vi "Graph - Multi-Y.vi"() -> ()   [LabVIEW 2013, in "Workspace MultiY Graph.lvlib"]
doc: "Sample numeric display item."
uses:
  Workspace MultiY Graph.lvlib
  <vilib>/NI Veristand/Display Template Support/Display Template Support.llb/cluster_Screen Item Settings.ctl
  <vilib>/NI Veristand/Display Template Support/Display Template Support.llb/cluster_Graph Scale Settings.ctl
  <vilib>/NI Veristand/Display Template Support/Display Template Support.llb/cluster_Graph Plot Settings.ctl
  NationalInstruments.VeriStand.SystemStorage
  XY Top level workspace graph data.ctl
  <vilib>/NI Veristand/Execution/Workspace/SystemStateRegEventRef.ctl
  <vilib>/NI Veristand/Display Template Support/Display Template Support.llb/enum_Display Template Handler Minimal To Widget Msg.ctl
  XY Dialog Msg to Control.ctl
  XY Dialog Msg Type.ctl
  XY Persistent Data.ctl
  XY Graph Properties.ctl
  XY Plot Properties.ctl
  XY Scale Properties.ctl
  XY Scale Precision.ctl
  XY Scale Format.ctl
  UDP Data.ctl
  Update Rate.ctl
  XY References.ctl
  <vilib>/NI Veristand/Display Template Support/Display Template Support.llb/enum_Display Template Handler Minimal To Workspace.ctl
  <vilib>/NI Veristand/Execution/Workspace/WorkspaceAPI.ctl
  <vilib>/NI Veristand/Execution/Workspace/SystemStateEventRef.ctl
  XY Control Msg to Dialog.ctl
  <vilib>/NI Veristand/UI Controls/Tree and Alias Browser/Net Event Data Ref.ctl
  <vilib>/NI Veristand/UI Controls/Tree and Alias Browser/Net Event Data.ctl
  <vilib>/NI Veristand/UI Controls/Tree and Alias Browser/Net Event.ctl
  <vilib>/NI Veristand/Execution/Workspace/UDPChannelStreamSession.ctl
  UDP Queue Data.ctl
  UDP Action State.ctl
  Graph Update Queue Data.ctl
  Graph Update Action State.ctl
  UDP Stream Configuration.ctl
  <vilib>/NI Veristand/Execution/Workspace/SystemState.ctl
  <vilib>/Utility/tcp.llb/UDP Multicast Read-Only Open.vi
  <vilib>/NI Veristand/Execution/Workspace/NI_VS Workspace ExecutionAPI.lvlib
  NationalInstruments.VeriStand.ClientAPI
  <vilib>/NI Veristand/UI Controls/Tree and Alias Browser/NI_VS UI Tree Alias Browser.lvlib
panel:
  in  "NIVS.Workspace Event":refnum<event-registration>
  in  "NIVS.System Definition Root":refnum<k24>
  in  "NIVS.Gateway IP Address":string
  out "Label":string="Waveform Graph"
  out "Graph":cluster{"X":dbl[], "Y":dbl[]}[](graph)
  in  "Item.Data":T1
  out "Y.Autoscale":bool
  in  "Y.Scale.Once":bool
  in  "Y.Scale.Auto":bool
  out "X.Autoscale":bool
  in  "X.Scale.Once":bool
  in  "X.Scale.Auto":bool
  in  "Legend":bool
  in  "Setup":bool
  in  "Hold":bool
  # "Autoscale X"
  # "Autoscale Y"
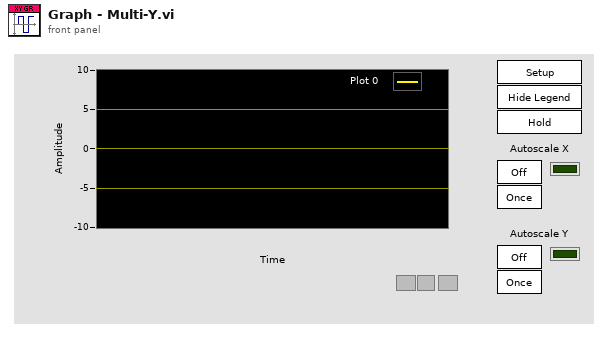
[diagram p1: front panel]
types:
  T1 = typedef "cluster_Screen Item Settings.ctl" = cluster{"Template VI":string, "Position X":i32, "Position Y":i32, "Custom":string, "Show Title Bar":bool, "ID":i32, "Always On Top":bool, "Allow Resize":bool, "Allow Minimize":bool, "Allow Close":bool, "Size to Screen":bool, "Screen.ID":i32, "State":enum16{"Normal", "New"}, "Title":string, "Window Bounds":cluster{"[0]":i16, "[1]":i16, "[2]":i16, "[3]":i16}, "Channel Ref":u64, "Unit":string, "Default Units?":bool, "Flash Limit?":bool, "Color 1":u32, "Color 2":u32, "Color 3":u32, "Color 4":u32, "Bck Color":u32, "Fore Color":u32, "Limit 1":dbl, "Limit 2":dbl, "Limit 3":dbl, "Limit 4":dbl, "Limit Mode 1":i32, "Limit Mode 2":i32, "Limit Mode 3":i32, "Limit Mode 4":i32, "Scale Precision":i32, "Scale Min":dbl, "Scale Max":dbl, "Format":i32, "Precision":i32, "Background Type":i32, "IDs":i32[], "Units":string[], "Labels":string[], "Scale Factor":dbl, "Scale Offset":dbl, "YScale Index":u32[], "XScale":T2, "YScales":T2[], "Plots":T3[], "Update Period":dbl, "History Length":dbl, "My.Ref":refnum<vi>, "Is Control?":bool, "Channel Paths":string[], "Custom Data":variant}
  T2 = typedef "cluster_Graph Scale Settings.ctl" = cluster{"Format":u8, "Precision":u8, "Fit":u8, "Label":string, "Use Default Label":bool, "Label Visible":bool, "Min":dbl, "Max":dbl}
  T3 = typedef "cluster_Graph Plot Settings.ctl" = cluster{"Bar Style":u8, "Fill To":i16, "Fill/PtColor":u32, "Line Style":u8, "Line Width":u8, "Color":u32, "Interp":u8, "Point Style":u8}
  T4 = typedef "Workspace MultiY Graph.lvlib/UDP Action State.ctl" = enum16{"Idle", "Open", "Acquire", "Send", "Close"}
  T5 = typedef "Workspace MultiY Graph.lvlib/UDP Stream Configuration.ctl" = cluster{"net address":u32, "Port":u16, "Channel IDs":i32[], "Packet IDs":i32[], "max packet size":i32, "Graph Buffer Size":i32, "Decimation":i32, "UDP Buffer Size":u32}
  T6 = cluster{"connection ID":refnum<k16>, "UDP Stream Configuration":T5, "Graph Buffer":cluster{"X":dbl[], "Y":dbl[]}[], "Dynamic VI Refs":refnum<vi>[]}
  T7 = typedef "Workspace MultiY Graph.lvlib/Graph Update Action State.ctl" = enum16{"Active", "Change Rate", "Inactive"}
  T8 = typedef "Workspace MultiY Graph.lvlib/Graph Update Queue Data.ctl" = cluster{"Graph Update Action State":T7, "Data":variant}
  T9 = typedef "Workspace MultiY Graph.lvlib/UDP Queue Data.ctl" = cluster{"UDP Action State":T4, "Data":variant}
  T10 = typedef "Workspace MultiY Graph.lvlib/XY Top level workspace graph data.ctl" = cluster{"Custom Data":variant, "EventRegs":cluster{"SystemChange":T11, "WorkspaceState":refnum<event-registration>, "Graph":refnum<event-registration>, "Wks&Dialog&Periodic":refnum<event-registration>}, "References":T12, "Persistent Data":T13, "System":cluster{"To Workspace":refnum<user-event>, "From Workspace":refnum<user-event>, "NIVS helper":refnum<vi>, "Gtwy":string, "Root":refnum<k24>, "Workspace":T21, "SystemStateRefs":T22, "Connected?":bool, "FromDialog":refnum<user-event>, "ErrFlag":bool, "New":bool, "ErrState":string, "Save":bool, "Hold":bool, "Periodic":refnum<user-event>, "ToDialog":refnum<user-event>, "DialogEventReg":refnum<event-registration>, "UseSavedWidth":bool, "TreeBrowserEventReg":refnum<event-registration>, "UDPChannelStreamSession":T23, "Valid Channels?":bool, "Update Graph":refnum<user-event>, "UDP Queue":refnum<queue>, "Graph Update Queue":refnum<queue>}, "GraphData":cluster{"X":dbl[], "Y":dbl[]}[], "UDP Stream Active?":bool}
  T11 = typedef "NI_VS Workspace ExecutionAPI.lvlib/SystemStateRegEventRef.ctl" = refnum<event-registration>
  T12 = typedef "Workspace MultiY Graph.lvlib/XY References.ctl" = cluster{"X.Scale.Auto":refnum<vi>, "Y.Scale.Auto":refnum<vi>, "X.Scale.Once":refnum<vi>, "Y.Scale.Once":refnum<vi>, "LegendVis":refnum<vi>, "Graph":refnum<vi>}
  T13 = typedef "Workspace MultiY Graph.lvlib/XY Persistent Data.ctl" = cluster{"Label":string, "Graph Props":T14, "UDP Data":T19}
  T14 = typedef "Workspace MultiY Graph.lvlib/XY Graph Properties.ctl" = cluster{"Plots":T15[], "Legend:Number of Rows":u32, "Scale Properties":T16, "Legend:Visible":bool, "BgColor":u32, "Last Plot Width":u32, "Resize":bool}
  T15 = typedef "Workspace MultiY Graph.lvlib/XY Plot Properties.ctl" = cluster{"Bar Plot Style":u8, "Digital Line Style":u8, "Digital Transition Location":u8, "Digital Transition Type":u8, "Fill To":i16, "Fill/Point Color":u32, "Label Format":u8, "Line Style":u8, "Line Width":u8, "Plot Color":u32, "Plot Interpolation":u8, "Point Style":u8, "Visible":bool, "X Scale Index":u32, "Y Scale Index":u32}
  T16 = typedef "Workspace MultiY Graph.lvlib/XY Scale Properties.ctl" = cluster{"X.Auto":bool, "X.Min":dbl, "X.Max":dbl, "X.IgnoreTS":bool, "X.Precision":T17, "X.Label:":string, "X.LabelVis":bool, "X.DefLabel":bool, "Y.Auto":bool, "Y.Min":dbl, "Y.Max":dbl, "Y.Format":T18, "Y.Precision:":T17, "Y.Label:":string, "Y.LabelVis":bool, "Y.DefLabel":bool, "X.Format":T18}
  T17 = typedef "Workspace MultiY Graph.lvlib/XY Scale Precision.ctl" = u8
  T18 = typedef "Workspace MultiY Graph.lvlib/XY Scale Format.ctl" = u8
  T19 = typedef "Workspace MultiY Graph.lvlib/UDP Data.ctl" = cluster{"Decimation":i32, "UDP Buffer Size":u32, "History Length":dbl, "Update Rate":T20, "Channel Paths":string[], "Channel Names":string[]}
  T20 = typedef "Workspace MultiY Graph.lvlib/Update Rate.ctl" = enum8{"15 Hz", "10 Hz", "5 Hz", "4 Hz", "3 Hz", "2 Hz", "1 Hz", "0.5 Hz"}
  T21 = typedef "NI_VS Workspace ExecutionAPI.lvlib/WorkspaceAPI.ctl" = refnum<k24>
  T22 = typedef "NI_VS Workspace ExecutionAPI.lvlib/SystemStateEventRef.ctl" = cluster{"CustDatRef":refnum<user-event>, "EvtRef":refnum<k27>}
  T23 = typedef "NI_VS Workspace ExecutionAPI.lvlib/UDPChannelStreamSession.ctl" = refnum<k24>
  T24 = cluster{"connection ID":refnum<k16>, "UDP Stream Configuration out":T5, "Array Out":cluster{"X":dbl[], "Y":dbl[]}[], "Dynamic VI Refs":refnum<vi>[]}
  T25 = typedef "Workspace MultiY Graph.lvlib/XY Control Msg to Dialog.ctl" = enum16{"Stop", "Connecting", "Disconnecting"}
  T26 = typedef "enum_Display Template Handler Minimal To Workspace.ctl" = cluster{"Operation":enum16{"SetCustomData", "DeleteItem"}, "Data":variant}
  T27 = cluster{"SystemChange":T11, "WorkspaceState":refnum<event-registration>, "Graph":refnum<event-registration>, "Wks&Dialog&Periodic":refnum<event-registration>}
  T28 = typedef "enum_Display Template Handler Minimal To Widget Msg.ctl" = enum16{"Stop", "LaunchConfigDialog"}
  T29 = typedef "Workspace MultiY Graph.lvlib/XY Dialog Msg Type.ctl" = enum16{"Update", "Delete"}
  T30 = typedef "NI_VS Workspace ExecutionAPI.lvlib/SystemState.ctl" = u8
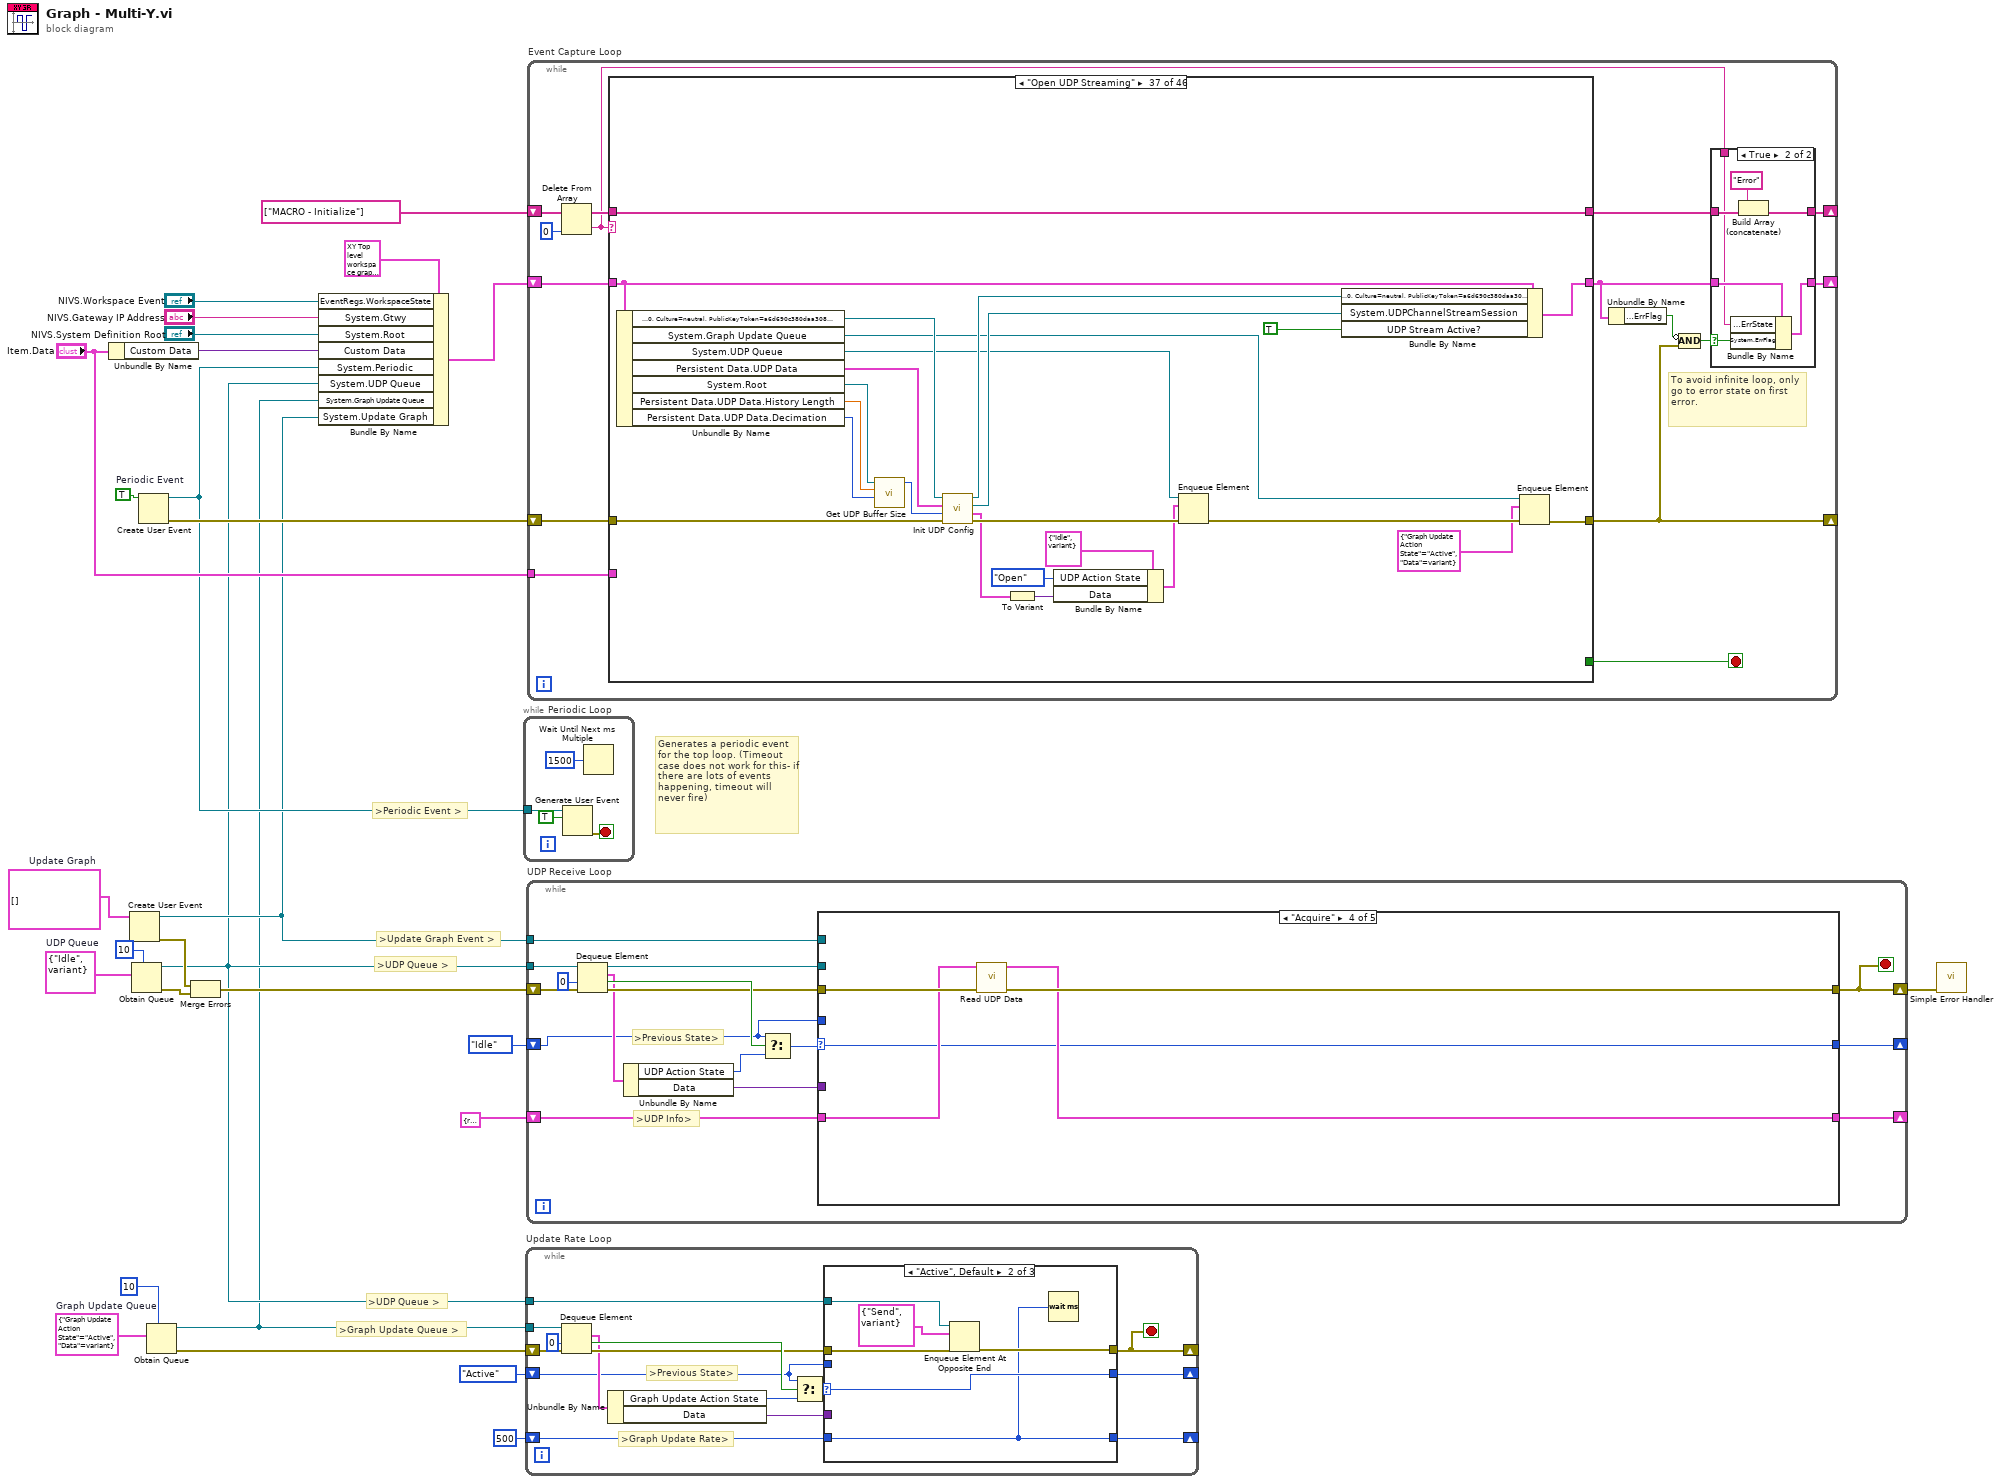
[diagram p0: block diagram]
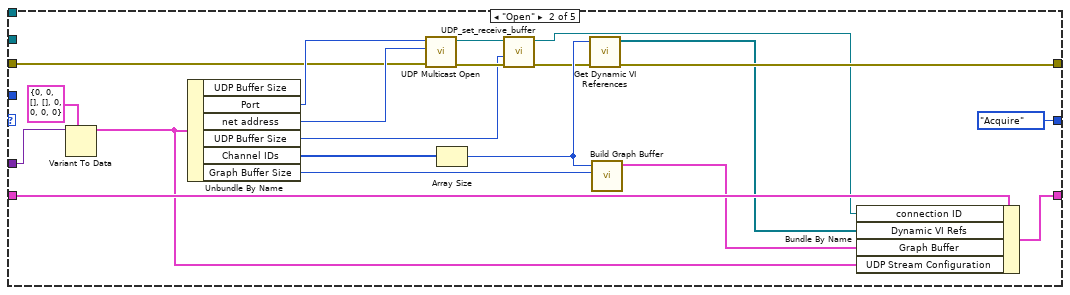
[diagram p3: hidden frame]
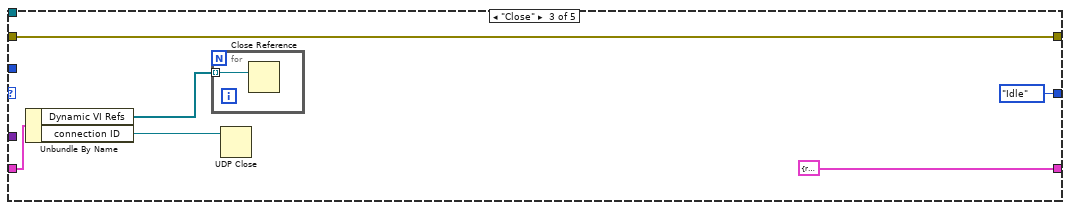
[diagram p4: hidden frame]
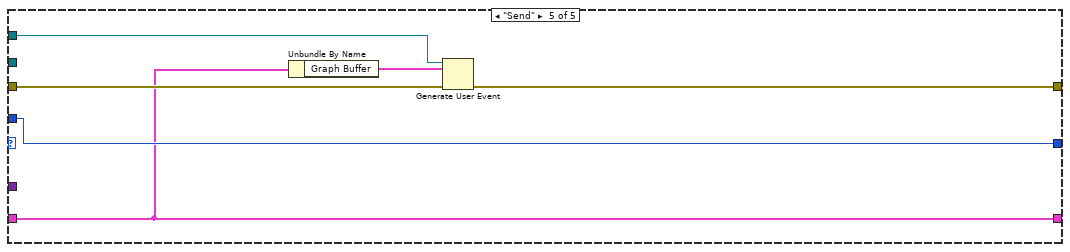
[diagram p5: hidden frame]
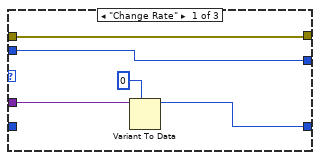
[diagram p6: hidden frame]
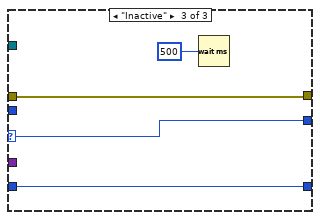
[diagram p7: hidden frame]
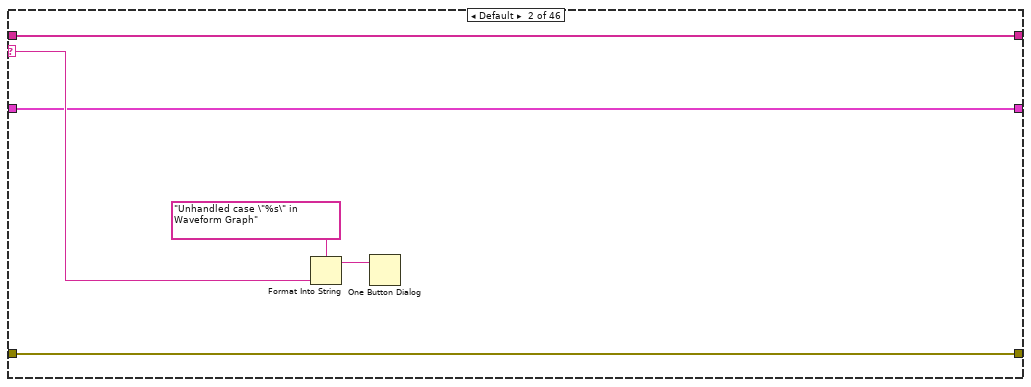
[diagram p10: hidden frame]
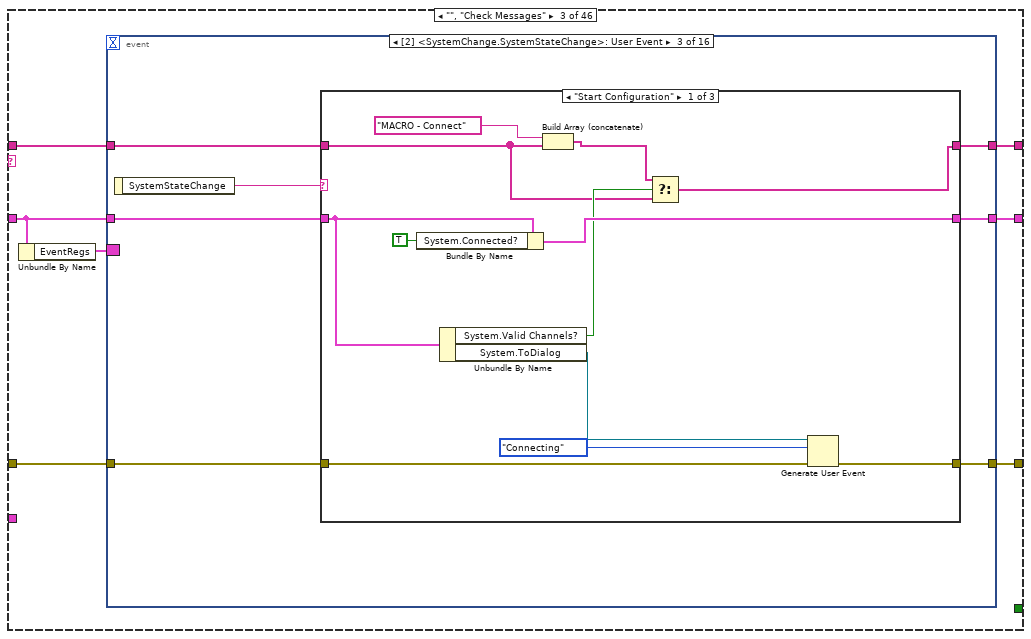
[diagram p11: hidden frame]
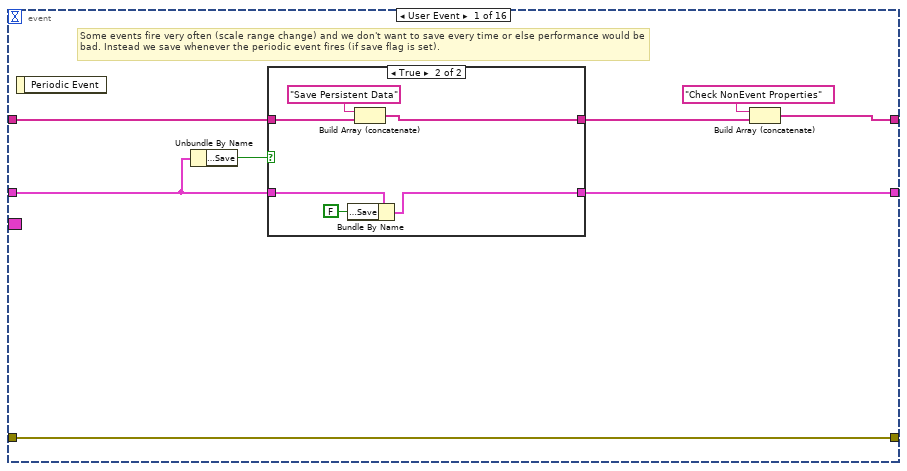
[diagram p12: hidden frame]
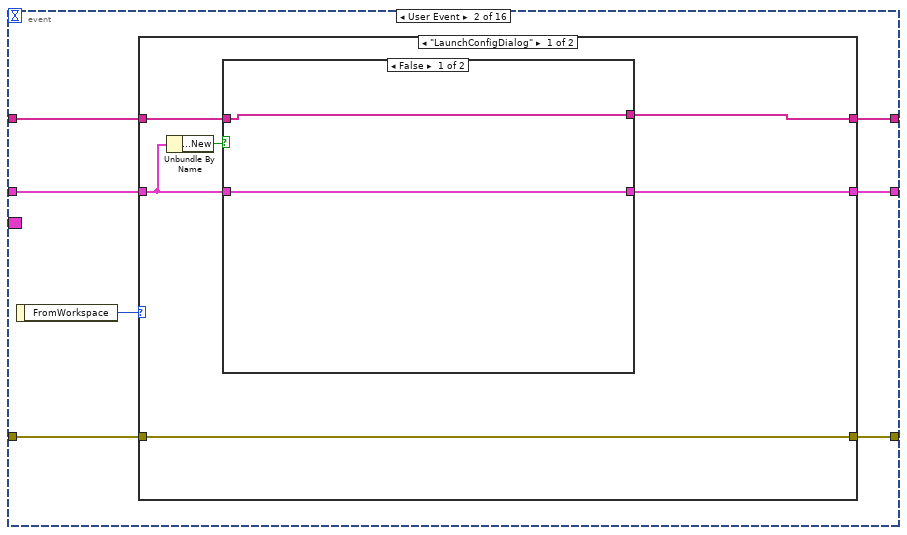
[diagram p14: hidden frame]
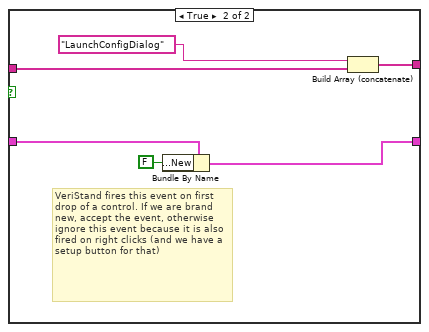
[diagram p15: hidden frame]
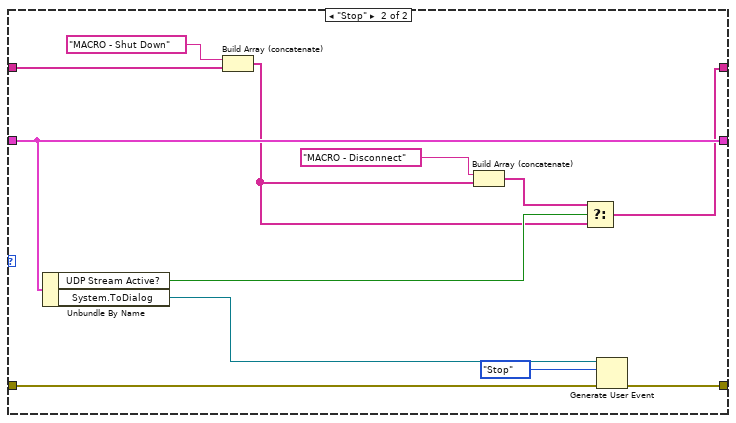
[diagram p16: hidden frame]
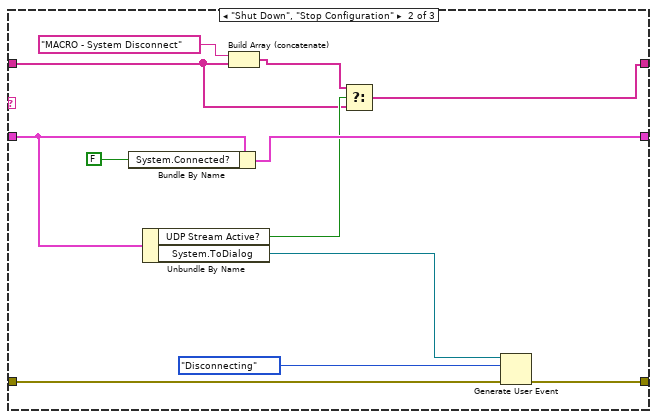
[diagram p17: hidden frame]
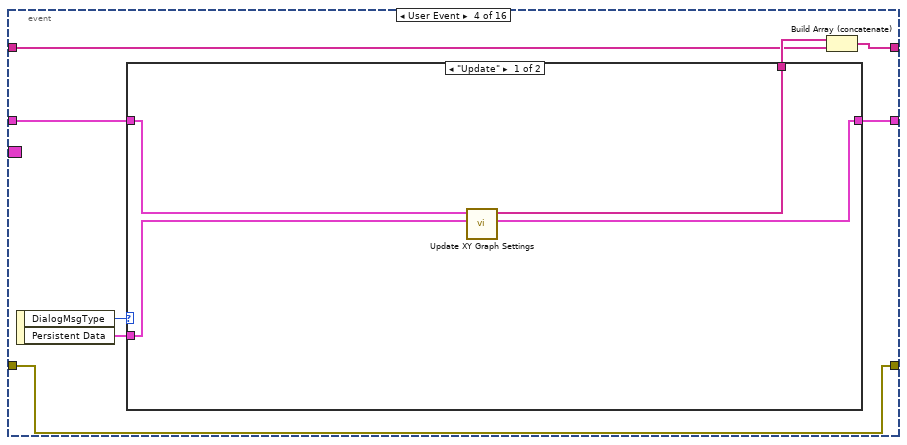
[diagram p19: hidden frame]
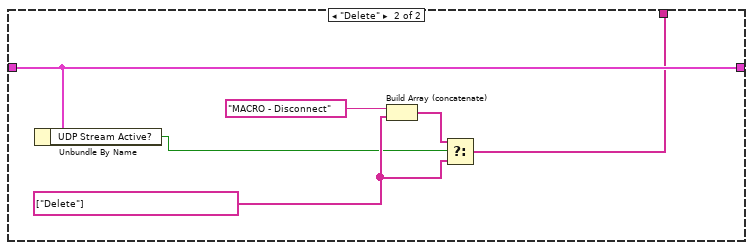
[diagram p20: hidden frame]
diagram:
  w14 = T8 {"Graph Update Action State"=enum."Active", "Data"=variant}  # Graph Update Queue
  w16 = T9 {"UDP Action State"=enum."Idle", "Data"=variant}  # UDP Queue
  w17 = cluster{"X":dbl[], "Y":dbl[]}[] []  # Update Graph
  w19 = TRUE  # Periodic Event
  # ">UDP Queue >"
  # ">Update Graph Event >"
  # ">Periodic Event >"
  # ">Graph Update Queue >"
  # ">UDP Queue >"
  # "Generates a periodic event for the top loop. (Timeout case does not work for this- if there are lots of events happening, timeout will never fire)"
  n1 = Unbundle By Name("Item.Data") -> ("Custom Data"=w27:variant)
  n2 = Create User Event(user event datatype=w17) -> (user event=w15:refnum<user-event>, error out=w10:errorcluster)  [unwired: 1 in]
  n3 = Obtain Queue(max queue size (-1, unlimited)=10, element data type=w16) -> (queue out=w7:refnum<queue>, error out=w11:errorcluster)  [unwired: 3 in, 1 out]
  n4 = Create User Event(user event datatype=w19) -> (user event=w18:refnum<user-event>, error out=w20:errorcluster)  [unwired: 1 in]
  n5 = Obtain Queue(max queue size (-1, unlimited)=10, element data type=w14) -> (queue out=w4:refnum<queue>, error out=w12:errorcluster)  [unwired: 3 in, 1 out]
  n6 = Merge Errors(w10, w11) -> (w9:errorcluster)
  n7 = Bundle By Name(cluster=T10 {"Custom Data"=variant, "EventRegs"={"SystemChange"=refnum, "WorkspaceState"=refnum, "Graph"=refnum, "Wks&Dialog&Periodic"=refnum}, "References"={"X.Scale.Auto"=refnum, "Y.Scale.Auto"=refnum, "X.Scale.Once"=refnum, "Y.Scale.Once"=refnum, "LegendVis"=refnum, "Graph"=refnum}, "Persistent Data"={"Label"="", "Graph Props"={"Plots"=[], "Legend:Number of Rows"=0, "Scale Properties"={"X.Auto"=FALSE, "X.Min"=0.0, "X.Max"=0.0, "X.IgnoreTS"=FALSE, "X.Precision"=0, "X.Label:"="", "X.LabelVis"=FALSE, "X.DefLabel"=FALSE, "Y.Auto"=FALSE, "Y.Min"=0.0, "Y.Max"=0.0, "Y.Format"=0, "Y.Precision:"=0, "Y.Label:"="", "Y.LabelVis"=FALSE, "Y.DefLabel"=FALSE, "X.Format"=0}, "Legend:Visible"=FALSE, "BgColor"=0, "Last Plot Width"=0, "Resize"=FALSE}, "UDP Data"={"Decimation"=0, "UDP Buffer Size"=0, "History Length"=0.0, "Update Rate"=enum."15 Hz", "Channel Paths"=[], "Channel Names"=[]}}, "System"={"To Workspace"=refnum, "From Workspace"=refnum, "NIVS helper"=refnum, "Gtwy"="", "Root"=refnum, "Workspace"=refnum, "SystemStateRefs"={"CustDatRef"=refnum, "EvtRef"=refnum}, "Connected?"=FALSE, "FromDialog"=refnum, "ErrFlag"=FALSE, "New"=FALSE, "ErrState"="", "Save"=FALSE, "Hold"=FALSE, "Periodic"=refnum, "ToDialog"=refnum, "DialogEventReg"=refnum, "UseSavedWidth"=FALSE, "TreeBrowserEventReg"=refnum, "UDPChannelStreamSession"=refnum, "Valid Channels?"=FALSE, "Update Graph"=refnum, "UDP Queue"=refnum, "Graph Update Queue"=refnum}, "GraphData"=[], "UDP Stream Active?"=FALSE} ("Waveform Graph Data"), "EventRegs.WorkspaceState"="NIVS.Workspace Event", "System.Gtwy"="NIVS.Gateway IP Address", "System.Root"="NIVS.System Definition Root", "Custom Data"=w27, "System.Periodic"=w18, "System.UDP Queue"=w7, "System.Graph Update Queue"=w4, "System.Update Graph"=w15) -> (w22:T10)
  n8 = while "Periodic Loop" {
    tunnel: w18 -> [w31]
    stop <- w30 stop-if-true
    n9 = Generate User Event(user event=w31, event data cluster=TRUE ("event data")) -> (error out=w30:errorcluster)  [unwired: 2 in, 1 out]
    n10 = Wait Until Next ms Multiple(millisecond multiple=u32 1500) -> ()  [unwired: 1 out]
  }
  n11 = while "Update Rate Loop" {
    tunnel: w4 -> [w46]
    shift-right: [w40] -> _
    shift-left: w12 -> [w47]
    shift-right: [w42] -> _
    shift-left: Graph_Update_Action_State."Active" ("Graph Update Action State") -> [w34]
    tunnel: w7 -> [w39]
    shift-right: [w35] -> _
    shift-left: u32 500 ("element") -> [w33]
    stop <- w40 stop-if-true
    # ">Previous State>"
    # ">Graph Update Rate>"
    n12 = Dequeue Element(queue=w46, timeout in ms (-1)=0, error in (no error)=w47) -> (element=w38:T8, timed out?=w44:bool, error out=w41:errorcluster)  [unwired: 1 out]
    n13 = Unbundle By Name(w38) -> ("Graph Update Action State"=w37:T7, "Data"=w36:variant)
    n14 = Select(t=w34, s=w44, f=w37) -> (s? t:f=w43:T7)
    n15 = case shown="\"Active\", Default" w43 {
      selector: w43 -> [_ w58 w62]
      tunnel: [w48 w58 w62] -> w42
      tunnel: w41 -> [w52 w57 w61]
      tunnel: [w52 w54 w61] -> w40
      tunnel: w39 -> [_ w56 _]
      tunnel: w36 -> [w51 _ _]
      tunnel: [w49 w53 w59] -> w35
      tunnel: w34 -> [w48 _ _]
      tunnel: w33 -> [_ w53 w59]
      frame "Change Rate" {
        n16 = Variant To Data(type=u32 0 ("element"), Variant=w51) -> (data=w49:u32)  [unwired: 1 in, 1 out]
      }
      frame "Active", Default {
        n17 = Enqueue Element At Opposite End(queue=w56, element=T9 {"UDP Action State"=enum."Send", "Data"=variant} ("notification"), error in (no error)=w57) -> (error out=w54:errorcluster)  [unwired: 1 in, 2 out]
        n18 = Wait (ms)(milliseconds to wait=w53) -> ()  [unwired: 1 out]
      }
      frame "Inactive" {
        n19 = Wait (ms)(milliseconds to wait=u32 500) -> ()  [unwired: 1 out]
      }
    }
  }
  n20 = while "UDP Receive Loop" {
    tunnel: w7 -> [w77]
    shift-right: [w71] -> w1
    shift-left: w9 -> [w78]
    shift-right: [w73] -> _
    shift-left: UDP_Action_State."Idle" ("UDP Action State") -> [w64]
    shift-right: [w69] -> _
    shift-left: T6 {"connection ID"=refnum, "UDP Stream Configuration"={"net address"=0, "Port"=0, "Channel IDs"=[], "Packet IDs"=[], "max packet size"=0, "Graph Buffer Size"=0, "Decimation"=0, "UDP Buffer Size"=0}, "Graph Buffer"=[], "Dynamic VI Refs"=[]} -> [w70]
    tunnel: w15 -> [w63]
    stop <- w71 stop-if-true
    # ">UDP Info>"
    # ">Previous State>"
    n21 = Dequeue Element(queue=w77, timeout in ms (-1)=0, error in (no error)=w78) -> (queue out=w76:refnum<queue>, element=w66:T9, timed out?=w74:bool, error out=w72:errorcluster)
    n22 = Unbundle By Name(w66) -> ("UDP Action State"=w67:T4, "Data"=w65:variant)
    n23 = Select(t=w64, s=w74, f=w67) -> (s? t:f=w68:T4)
    n24 = case shown="\"Acquire\"" w68 {
      selector: w68 -> [w81 _ _ w109 _]
      tunnel: w72 -> [w80 w89 w103 w113 w116]
      tunnel: [w80 w94 w103 w112 w115] -> w71
      tunnel: w76 -> [_ _ _ _ _]
      tunnel: [w81 UDP_Action_State."Acquire" ("UDP Action State") UDP_Action_State."Idle" ("UDP Action State") w109 w119] -> w73
      tunnel: w70 -> [w79 w98 w106 w111 w114]
      tunnel: [w79 w97 T24 {"connection ID"=refnum, "UDP Stream Configuration out"={"net address"=0, "Port"=0, "Channel IDs"=[], "Packet IDs"=[], "max packet size"=0, "Graph Buffer Size"=0, "Decimation"=0, "UDP Buffer Size"=0}, "Array Out"=[], "Dynamic VI Refs"=[]} w110 w114] -> w69
      tunnel: w65 -> [_ w92 _ _ _]
      tunnel: w64 -> [_ _ _ _ w119]
      tunnel: w63 -> [_ _ _ _ w117]
      frame "Idle", Default {
      }
      frame "Open" {
        n25 = Variant To Data(type=T5 {"net address"=0, "Port"=0, "Channel IDs"=[], "Packet IDs"=[], "max packet size"=0, "Graph Buffer Size"=0, "Decimation"=0, "UDP Buffer Size"=0} ("UDP Stream Configuration out"), Variant=w92) -> (data=w90:T5)  [unwired: 1 in, 1 out]
        n26 = Unbundle By Name(w90) -> ("Port"=w101:u16, "net address"=w100:u32, "UDP Buffer Size"=w82:u32, "Channel IDs"=w96:i32[], "Graph Buffer Size"=w99:i32)  [unwired: 1 out]
        n27 = call-poly <vilib>:"UDP Multicast Open.vi"("error in (no error)"=w89, "multicast addr"=w100, "port"=w101) -> ("error out"=w86:errorcluster, "connection ID"=w85:refnum<k16>)  [unwired: 6 in, 1 out]
        n28 = Array Size(array=w96) -> (size(s)=w95:i32)
        n29 = call "UDP_set_receive_buffer.vi"("error in (no error)"=w86, "Receive Buffer Size"=w82, "connection ID"=w85) -> ("error out"=w83:errorcluster, "connection ID out"=w84:refnum<k16>)  [unwired: 6 in]
        n30 = call "Get Dynamic VI References.vi"("error in (no error)"=w83, "Channel Count"=w95) -> ("error out"=w94:errorcluster, "Dynamic VI References"=w93:refnum<vi>[])  [unwired: 8 in]
        n31 = call "Build Graph Buffer.vi"("Graph Buffer Size"=w99, "Channel Count"=w95) -> ("Graph Buffer out"=w87:cluster{dbl[], dbl[]}[])  [unwired: 9 in]
        n32 = Bundle By Name(cluster=w98, "connection ID"=w84, "Dynamic VI Refs"=w93, "Graph Buffer"=w87, "UDP Stream Configuration"=w90) -> (w97:T6)
      }
      frame "Close" {
        n33 = Unbundle By Name(w106) -> ("Dynamic VI Refs"=w105:refnum<vi>[], "connection ID"=w104:refnum<k16>)
        n34 = for {
          tunnel: w105 -> [w108] mode=indexing
          n35 = Close Reference(reference=w108) -> ()  [unwired: 1 in, 1 out]
        }
        n36 = UDP Close(connection ID=w104) -> ()  [unwired: 1 in, 2 out]
      }
      frame "Acquire" {
        n37 = call "Read UDP Data.vi"("error in (no error)"=w113, "UDP Cluster in"=w111) -> ("error out"=w112:errorcluster, "UDP Cluster out"=w110:T6)  [unwired: 8 in]
      }
      frame "Send" {
        n38 = Unbundle By Name(w114) -> ("Graph Buffer"=w118:cluster{"X":dbl[], "Y":dbl[]}[])
        n39 = Generate User Event(user event=w117, event data cluster=w118, error in=w116) -> (error out=w115:errorcluster)  [unwired: 1 in, 1 out]
      }
    }
  }
  n40 = while "Event Capture Loop" {
    shift-right: [w128] -> _
    shift-left: string[] ["MACRO - Initialize"] -> [w134]
    shift-right: [w121] -> _
    shift-left: w20 -> [w127]
    shift-right: [w125] -> _
    shift-left: w22 -> [w130]
    tunnel: "Item.Data" -> [w129]
    stop <- w132 stop-if-true
    # "To avoid infinite loop, only go to error state on first error."
    n41 = Delete From Array(array=w134, index=0) -> (deleted portion=w120:string, array with subset deleted=w133:string[])  [unwired: 1 in]
    n42 = case shown="\"Open UDP Streaming\"" w120 {
      selector: w120 -> [_ w151 _ _ _ _ _ _ _ _ _ _ _ _ _ _ _ _ _ _ _ _ _ _ _ _ _ _ _ _ _ _ _ _ _ _ _ _ _ _ _ _ _ _ _ _]
      tunnel: [w144 w147 w159 string[] ["MACRO - Disconnect"] w442 w450 w452 w461 w462 w472 w484 w487 w491 w509 w532 w543 w554 w587 w621 w637 w658 w683 w691 w701 w702 w706 w709 w716 w720 w725 w730 w735 w741 w757 w771 w774 w798 w799 w808 w811 w820 w825 w840 w849 w873 w891] -> w131
      tunnel: w133 -> [w144 w147 w158 _ w442 w450 w452 w461 w462 w472 w484 w487 w491 w509 w532 w543 w554 w587 w621 w637 w658 w683 w691 w701 w702 w706 w710 w717 w723 w726 w731 w738 w741 w757 w771 w774 w798 w799 w808 w811 w820 w829 w840 w848 w873 w891]
      tunnel: [_ _ _ _ _ _ _ _ _ _ _ _ _ _ _ _ _ _ _ _ _ _ _ _ TRUE _ _ _ _ _ _ _ _ _ _ _ _ _ _ _ _ _ _ _ _ _] -> w132
      tunnel: w127 -> [w146 w149 w156 w426 w438 w449 w454 w455 w468 w471 w475 w486 w490 w508 w531 w542 w549 w586 w620 w634 w660 w669 w690 w694 w704 w708 w713 w718 w722 w728 w733 w737 w740 w754 w768 w773 w796 w801 w807 w810 w823 w834 w839 w854 w871 w887]
      tunnel: [w146 w149 w155 errorcluster {"status"=FALSE, "code"=0, "source"=""} ("error constant") w441 w446 w453 w455 w466 w471 w474 w486 w490 w497 w519 w539 w550 w578 w617 w635 w660 w676 w687 w693 w704 w708 w713 w718 w722 w728 w733 w737 w740 w743 w760 w773 w789 w801 w802 w812 w823 w833 w839 w853 w867 w888] -> w121
      tunnel: w130 -> [w145 w148 w154 w428 w435 w448 w451 w460 w469 w470 w483 w485 w489 w501 w524 w541 w553 w585 w619 w636 w659 w686 w689 w700 w703 w707 w712 w715 w721 w727 w732 w736 w739 w753 w767 w772 w793 w800 w804 w809 w822 w831 w838 w844 w872 w881]
      tunnel: [w145 w148 w157 w428 w434 w447 w451 w459 w469 w470 w483 w485 w489 w500 w523 w541 w553 w585 w619 w636 w659 w686 w689 w700 w703 w707 w712 w715 w721 w727 w732 w736 w739 w752 w766 w772 w792 w800 w806 w813 w821 w830 w837 w846 w872 w875] -> w124
      tunnel: w129 -> [_ _ _ _ _ _ _ _ _ _ _ _ _ _ _ _ _ _ _ _ _ _ _ _ _ _ _ _ _ _ _ _ _ _ _ _ _ _ _ _ _ _ _ _ _ w877]
      frame "<------------------ System ------------------>" {
      }
      frame Default {
        n43 = Format Into String(format string="Unhandled case \"%s\" in Waveform Graph", w151) -> (resulting string=w152:string)  [unwired: 2 in, 1 out]
        n44 = One Button Dialog(message=w152) -> ()  [unwired: 1 in, 1 out]
      }
      frame "", "Check Messages" {
        n45 = Unbundle By Name(w154) -> ("EventRegs"=w153:T27)
        n46 = event shown="[2] <SystemChange.SystemStateChange>: User Event" {
          selector: w153 -> [_ _ _ _ _ _ _ _ _ _ _ _ _ _ _ _]
          dyn-events: _ -> [_ _ _ _ _ _ _ _ _ _ _ _ _ _ _ _]
          timeout: _ -> [_ _ _ _ _ _ _ _ _ _ _ _ _ _ _ _]
          tunnel: [w160 w176 w215 w248 w267 w288 w295 w302 w308 w318 w325 w337 w345 w356 w369 w382] -> w159
          tunnel: w158 -> [w167 w180 w214 w249 w266 w288 w295 w304 w316 w323 w330 w340 w351 w362 w369 w381]
          tunnel: [w166 w177 w213 w247 w265 w286 w291 w306 w310 w320 w327 w339 w343 w354 w364 w383] -> w157
          tunnel: w154 -> [w164 w178 w212 w246 w264 w283 w294 w306 w312 w321 w328 w333 w348 w359 w367 w384]
          tunnel: w156 -> [w163 w182 w210 w243 w262 w284 w293 w305 w315 w322 w329 w335 w350 w361 w368 w385]
          tunnel: [w163 w179 w211 w243 w263 w284 w292 w305 w314 w322 w329 w334 w349 w360 w368 w386] -> w155
          event User Event {
            # "Some events fire very often (scale range change) and we don't want to save every time or else performance would be bad. Instead we save whenever the periodic event fires (if save flag is set)."
            n47 = event-data() -> ()  [unwired: 1 in, 1 out]
            n48 = Unbundle By Name(w164) -> ("System.Save"=w165:bool)
            n49 = case shown="True" w165 {
              tunnel: w167 -> [w169 w172]
              tunnel: [w169 w170] -> w162
              tunnel: [w168 w173] -> w166
              tunnel: w164 -> [w168 w175]
              frame False {
              }
              frame True {
                n50 = Bundle By Name(cluster=w175, "System.Save"=FALSE) -> (w173:T10)
                n51 = Build Array (concatenate)("Save Persistent Data", w172) -> (w170:string[])
              }
            }
            n52 = Build Array (concatenate)("Check NonEvent Properties", w162) -> (w160:string[])
          }
          event User Event {
            n53 = event-data() -> ("FromWorkspace"=w181:T28)  [unwired: 1 in]
            n54 = case shown="\"LaunchConfigDialog\"" w181 {
              tunnel: w182 -> [w188 w205]
              tunnel: w180 -> [w187 w208]
              tunnel: [w188 w204] -> w179
              tunnel: w178 -> [w184 w206]
              tunnel: [w183 w206] -> w177
              tunnel: [w186 w197] -> w176
              frame "LaunchConfigDialog" {
                n55 = Unbundle By Name(w184) -> ("System.New"=w185:bool)
                n56 = case shown="False" w185 {
                  tunnel: w187 -> [w189 w196]
                  tunnel: [w189 w194] -> w186
                  tunnel: w184 -> [w190 w193]
                  tunnel: [w190 w192] -> w183
                  frame False {
                  }
                  frame True {
                    # "VeriStand fires this event on first drop of a control. If we are brand new, accept the event, otherwise ignore this event because it is also fired on right clicks (and we have a setup button for that)"
                    n57 = Bundle By Name(cluster=w193, "System.New"=FALSE) -> (w192:T10)
                    n58 = Build Array (concatenate)("LaunchConfigDialog", w196) -> (w194:string[])
                  }
                }
              }
              frame "Stop" {
                n59 = Unbundle By Name(w206) -> ("UDP Stream Active?"=w199:bool, "System.ToDialog"=w203:refnum<user-event>)
                n60 = Build Array (concatenate)("MACRO - Shut Down", w208) -> (w198:string[])
                n61 = Build Array (concatenate)("MACRO - Disconnect", w198) -> (w200:string[])
                n62 = Select(t=w200, s=w199, f=w198) -> (s? t:f=w197:string[])
                n63 = Generate User Event(user event=w203, event data cluster=XY_Control_Msg_to_Dialog."Stop" ("event data"), error in=w205) -> (error out=w204:errorcluster)  [unwired: 1 in, 1 out]
              }
            }
          }
          event User Event {
            n64 = event-data() -> ("SystemStateChange"=w209:string)  [unwired: 1 in]
            n65 = case shown="\"Start Configuration\"" w209 {
              tunnel: [w216 w228 w242] -> w215
              tunnel: w214 -> [w218 w229 w242]
              tunnel: [w226 w238 w241] -> w213
              tunnel: w212 -> [w221 w232 w241]
              tunnel: [w222 w233 w240] -> w211
              tunnel: w210 -> [w223 w234 w240]
              frame "Start Configuration" {
                n66 = Bundle By Name(cluster=w221, "System.Connected?"=TRUE) -> (w226:T10)
                n67 = Unbundle By Name(w221) -> ("System.Valid Channels?"=w219:bool, "System.ToDialog"=w225:refnum<user-event>)
                n68 = Build Array (concatenate)("MACRO - Connect", w218) -> (w217:string[])
                n69 = Select(t=w217, s=w219, f=w218) -> (s? t:f=w216:string[])
                n70 = Generate User Event(user event=w225, event data cluster=XY_Control_Msg_to_Dialog."Connecting" ("event data"), error in=w223) -> (error out=w222:errorcluster)  [unwired: 1 in, 1 out]
              }
              frame "Shut Down", "Stop Configuration" {
                n71 = Bundle By Name(cluster=w232, "System.Connected?"=FALSE) -> (w238:T10)
                n72 = Unbundle By Name(w232) -> ("UDP Stream Active?"=w231:bool, "System.ToDialog"=w236:refnum<user-event>)
                n73 = Build Array (concatenate)("MACRO - System Disconnect", w229) -> (w230:string[])
                n74 = Select(t=w230, s=w231, f=w229) -> (s? t:f=w228:string[])
                n75 = Generate User Event(user event=w236, event data cluster=XY_Control_Msg_to_Dialog."Disconnecting" ("event data"), error in=w234) -> (error out=w233:errorcluster)  [unwired: 1 in, 1 out]
              }
              frame Default {
              }
            }
          }
          event User Event {
            n76 = event-data() -> ("DialogMsgType"=w244:T29, "Persistent Data"=w245:T13)  [unwired: 1 in]
            n77 = case shown="\"Update\"" w244 {
              tunnel: w246 -> [w253 w260]
              tunnel: [w254 w260] -> w247
              tunnel: w245 -> [w252 _]
              tunnel: [w251 w256] -> w250
              frame "Update" {
                n78 = call "Update XY Graph Settings.vi"("Persistent Data"=w252, "Waveform Graph Data in"=w253) -> ("Waveform Graph Data out"=w254:T10, "State Array"=w251:string[])  [unwired: 8 in]
              }
              frame "Delete" {
                w258 = string[] ["Delete"]
                n79 = Unbundle By Name(w260) -> ("UDP Stream Active?"=w255:bool)
                n80 = Build Array (concatenate)("MACRO - Disconnect", w258) -> (w257:string[])
                n81 = Select(t=w257, s=w255, f=w258) -> (s? t:f=w256:string[])
              }
            }
            n82 = Build Array (concatenate)(w250, w249) -> (w248:string[])
          }
          event User Event {
            # "Workspace and/or project  is closing"
            n83 = event-data() -> ("Workspace Event"=w261:string)  [unwired: 1 in]
            n84 = case shown="\"Shut Down\"" w261 {
              tunnel: [w268 w282] -> w267
              tunnel: w266 -> [w279 w282]
              tunnel: [w273 w281] -> w265
              tunnel: w264 -> [w273 w281]
              tunnel: [w274 w280] -> w263
              tunnel: w262 -> [w275 w280]
              frame "Shut Down" {
                n85 = Unbundle By Name(w273) -> ("UDP Stream Active?"=w272:bool, "System.ToDialog"=w277:refnum<user-event>)
                n86 = Build Array (concatenate)("MACRO - Shut Down", w279) -> (w269:string[])
                n87 = Build Array (concatenate)("MACRO - System Disconnect", w269) -> (w270:string[])
                n88 = Select(t=w270, s=w272, f=w269) -> (s? t:f=w268:string[])
                n89 = Generate User Event(user event=w277, event data cluster=XY_Control_Msg_to_Dialog."Stop" ("event data"), error in=w275) -> (error out=w274:errorcluster)  [unwired: 1 in, 1 out]
              }
              frame Default {
              }
            }
          }
          event User Event {
            n90 = event-data() -> ("Update Graph"=w287:cluster{"X":dbl[], "Y":dbl[]}[])  [unwired: 1 in]
            n91 = Unbundle By Name(w283) -> ("System.Hold"=w285:bool)
            n92 = case shown="False" w285 {
              tunnel: w287 -> [w289 _]
              frame False {
                "Graph" <- w289
              }
              frame True {
              }
            }
            n93 = Bundle By Name(cluster=w283, "GraphData"=w287) -> (w286:T10)
          }
          event "Hold": Value Change {
            n94 = event-data() -> ("NewVal"=w290:bool)  [unwired: 1 in]
            n95 = case shown="False" w290 {
              tunnel: w294 -> [w300 _]
              tunnel: w293 -> [w299 w301]
              tunnel: [w298 w301] -> w292
              frame False {
                # "Graph was unheld. immediately refresh."
                n96 = Unbundle By Name(w300) -> ("References.Graph"=w297:refnum<vi>, "GraphData"=w296:cluster{"X":dbl[], "Y":dbl[]}[])
                n97 = property class="XYGraph (strict)"(reference=w297, error in=w299, "Value"=w296) -> (error out=w298:errorcluster)  [unwired: 1 out]
              }
              frame True {
                # "Graph held. The wfm data event case will not update the graph"
              }
            }
            n98 = Bundle By Name(cluster=w294, "System.Hold"=w290) -> (w291:T10)
          }
          event "Setup": Value Change {
            n99 = event-data() -> ()  [unwired: 1 in, 2 out]
            n100 = Build Array (concatenate)("LaunchConfigDialog", w304) -> (w302:string[])
          }
          event "Graph": Plot Attribute Change {
            # "Rather than figure out what changed exactly.. just read & save it all"
            n101 = event-data() -> ()  [unwired: 1 in, 1 out]
            n102 = Unbundle By Name(w312) -> ("References.Graph"=w313:refnum<vi>)
            n103 = call "Get XY Plot Properties from Graph.vi"("error in (no error)"=w315, "Graph"=w313) -> ("error out"=w314:errorcluster, "Plots"=w311:T15[], "Legend:Number of Rows"=w309:u32)  [unwired: 7 in]
            n104 = Build Array (concatenate)("Save Persistent Data", w316) -> (w308:string[])
            n105 = Bundle By Name(cluster=w312, "Persistent Data.Graph Props.Legend:Number of Rows"=w309, "Persistent Data.Graph Props.Plots"=w311) -> (w310:T10)
          }
          event "X.Scale.Auto": Value Change {
            n106 = event-data() -> ("NewVal"=w319:bool)  [unwired: 1 in]
            n107 = Bundle By Name(cluster=w321, "Persistent Data.Graph Props.Scale Properties.X.Auto"=w319) -> (w320:T10)
            n108 = Build Array (concatenate)(string[] ["Set Autoscale X", "Save Persistent Data"], w323) -> (w318:string[])
          }
          event "Y.Scale.Auto": Value Change {
            n109 = event-data() -> ("NewVal"=w326:bool)  [unwired: 1 in]
            n110 = Bundle By Name(cluster=w328, "Persistent Data.Graph Props.Scale Properties.Y.Auto"=w326) -> (w327:T10)
            n111 = Build Array (concatenate)(string[] ["Set Autoscale Y", "Save Persistent Data"], w330) -> (w325:string[])
          }
          event "Legend": Value Change {
            # "Handle here since it is only set here"
            n112 = event-data() -> ("NewVal"=w338:bool)  [unwired: 1 in]
            n113 = Unbundle By Name(w333) -> ("References.Graph"=w332:refnum<vi>)
            n114 = Not(x=w338) -> (.not. x?=w331:bool)
            n115 = property on="Property Node" class="XYGraph (strict)"(reference=w332, error in=w335, "Legend Visible"=w331) -> (error out=w334:errorcluster)  [unwired: 1 out]
            n116 = Bundle By Name(cluster=w333, "Persistent Data.Graph Props.Legend:Visible"=w331) -> (w339:T10)
            n117 = Build Array (concatenate)("Save Persistent Data", w340) -> (w337:string[])
          }
          event "Y.Scale.Once": Value Change {
            # "Handle here since this can only be called by the button and it is not persistent"
            n118 = event-data() -> ()  [unwired: 1 in, 1 out]
            n119 = Unbundle By Name(w348) -> ("References.Graph"=w347:refnum<vi>)
            n120 = property on="Property Node" class="XYGraph (strict)"(reference=w347, error in=w350, "YScale.ScaleFit"=u8 1 ("X Scale.Scale Fit")) -> (error out=w349:errorcluster, "YScale.Maximum"=w342:dbl, "YScale.Minimum"=w341:dbl)  [unwired: 1 out]
            n121 = Build Array (concatenate)("Save Persistent Data", w351) -> (w345:string[])
            n122 = Bundle By Name(cluster=w348, "Persistent Data.Graph Props.Scale Properties.Y.Max"=w342, "Persistent Data.Graph Props.Scale Properties.Y.Min"=w341) -> (w343:T10)
          }
          event "X.Scale.Once": Value Change {
            # "Handle here since this can only be called by the button and it is not persistent"
            n123 = event-data() -> ()  [unwired: 1 in, 1 out]
            n124 = Unbundle By Name(w359) -> ("References.Graph"=w358:refnum<vi>)
            n125 = property on="Property Node" class="XYGraph (strict)"(reference=w358, error in=w361, "XScale.ScaleFit"=u8 1 ("X Scale.Scale Fit")) -> (error out=w360:errorcluster, "XScale.Maximum"=w353:dbl, "XScale.Minimum"=w352:dbl)  [unwired: 1 out]
            n126 = Build Array (concatenate)("Save Persistent Data", w362) -> (w356:string[])
            n127 = Bundle By Name(cluster=w359, "Persistent Data.Graph Props.Scale Properties.X.Max"=w353, "Persistent Data.Graph Props.Scale Properties.X.Min"=w352) -> (w354:T10)
          }
          event "Graph": Scale Range Change {
            # "User changed scale manually"
            n128 = event-data() -> ("Kind"=w363:enum16{"X-Scale", "Y-Scale", "Z-Scale"}, "NewRange.Minimum"=w366:dbl, "NewRange.Maximum"=w365:dbl)  [unwired: 1 in]
            n129 = case shown="\"Y-Scale\"" w363 {
              tunnel: w367 -> [w374 w379 w380]
              tunnel: w366 -> [w373 w378 _]
              tunnel: w365 -> [w372 w377 _]
              tunnel: [w371 w376 w380] -> w364
              frame "Y-Scale" {
                n130 = Bundle By Name(cluster=w374, "Persistent Data.Graph Props.Scale Properties.Y.Min"=w373, "Persistent Data.Graph Props.Scale Properties.Y.Max"=w372, "System.Save"=TRUE) -> (w371:T10)
              }
              frame "X-Scale" {
                n131 = Bundle By Name(cluster=w379, "Persistent Data.Graph Props.Scale Properties.X.Min"=w378, "Persistent Data.Graph Props.Scale Properties.X.Max"=w377, "System.Save"=TRUE) -> (w376:T10)
              }
              frame Default {
              }
            }
          }
          event "Graph": Shortcut Menu Selection? (App) {
            n132 = event-data() -> ("ItemTag"=w387:string)  [unwired: 1 in]
            n133 = case shown="\"APP_SC_IGNORE_TIME_STAMP\"" w387 {
              tunnel: [FALSE ("Discard?") TRUE ("Discard?") TRUE ("Discard?") TRUE ("Discard?")] -> w388
              tunnel: [w389 w401 w412 w422] -> w386
              tunnel: w385 -> [w389 w402 w413 w423]
              tunnel: w384 -> [w391 w403 w411 w421]
              tunnel: [w391 w399 w411 w421] -> w383
              tunnel: [w390 w394 w409 w419] -> w382
              tunnel: w381 -> [w390 w395 w409 w419]
              frame Default {
              }
              frame "APP_SC_IGNORE_TIME_STAMP" {
                n134 = Unbundle By Name(w403) -> ("References.Graph"=w400:refnum<vi>)
                n135 = property class="XYGraph (strict)"(reference=w400, error in=w402) -> (error out=w401:errorcluster, "IgnoreTimestamp"=w398:bool)  [unwired: 1 out]
                n136 = Not(x=w398) -> (.not. x?=w397:bool)
                n137 = Build Array (concatenate)(string[] ["Set X&Y Format & Precision", "Save Persistent Data"], w395) -> (w394:string[])
                n138 = Bundle By Name(cluster=w403, "Persistent Data.Graph Props.Scale Properties.X.IgnoreTS"=w397) -> (w399:T10)
              }
              frame "APP_SC_AUTOSCALE_Y" {
                # "reroute it like a button press"
                n139 = Unbundle By Name(w411) -> ("References.Y.Scale.Auto"=w408:refnum<vi>)
                n140 = property class="Bool (strict)"(reference=w408, error in=w413) -> (reference out=w406:refnum<vi>, error out=w407:errorcluster, "Value"=w405:bool)
                n141 = Not(x=w405) -> (.not. x?=w404:bool)
                n142 = property class="Bool (strict)"(reference=w406, error in=w407, "Val(Sgnl)"=w404) -> (error out=w412:errorcluster)  [unwired: 1 out]
              }
              frame "APP_SC_AUTOSCALE_X" {
                # "reroute it like a button press"
                n143 = Unbundle By Name(w421) -> ("References.X.Scale.Auto"=w418:refnum<vi>)
                n144 = property class="Bool (strict)"(reference=w418, error in=w423) -> (reference out=w416:refnum<vi>, error out=w417:errorcluster, "Value"=w415:bool)
                n145 = Not(x=w415) -> (.not. x?=w414:bool)
                n146 = property class="Bool (strict)"(reference=w416, error in=w417, "Val(Sgnl)"=w414) -> (error out=w422:errorcluster)  [unwired: 1 out]
              }
            }
            n147 = event-data("Discard?"=w388) -> ()  [unwired: 1 in, 1 out]
          }
        }
      }
      frame "Error" {
        n148 = Unbundle By Name(w428) -> ("System.ErrState"=w427:string)
        n149 = Unbundle By Name(w426) -> ("source"=w430:string)
        n150 = Concatenate Strings(w430, "<APPEND> State: " ("string"), w427) -> (w425:string)
        n151 = Bundle By Name(cluster=w426, "source"=w425) -> (w424:errorcluster)
        n152 = call <vilib>:"Simple Error Handler.vi"("error in (no error)"=w424) -> ()  [unwired: 4 in, 5 out]
      }
      frame "Save Persistent Data" {
        # "Instead of calling once at shut down, this is called often. Because by the time we are shutting down, it is too late to save data- The workspace isnt listening."
        n153 = Unbundle By Name(w435) -> ("Persistent Data"=w436:T13)
        n154 = call "XY Persistent Data to Variant.vi"("error in (no error)"=w438, "Persistent Data"=w436) -> ("error out"=w437:errorcluster, "Variant"=w433:variant)  [unwired: 8 in]
        n155 = Bundle By Name(cluster=w435, "Custom Data"=w433) -> (w434:T10)
        n156 = Unbundle By Name(w434) -> ("System.To Workspace"=w445:refnum<user-event>, "Custom Data"=w440:variant)
        n157 = Bundle By Name(cluster=T26 {"Operation"=enum."SetCustomData", "Data"=variant} ("event data"), "Operation"=enum16{"SetCustomData", "DeleteItem"}."SetCustomData", "Data"=w440) -> (w443:T26)
        n158 = Generate User Event(user event=w445, event data cluster=w443, error in=w437) -> (error out=w441:errorcluster)  [unwired: 1 in, 1 out]
      }
      frame "Check NonEvent Properties" {
        # "use this case to check any properties that don't have an event associated with them. for example, someone changing a legend text doesn't fire an event... but we still want to save that change"
        n159 = call "Check For XY Renamed Plots.vi"("error in (no error)"=w449, "Waveform Graph Data in"=w448) -> ("error out"=w446:errorcluster, "Waveform Graph Data out"=w447:T10)  [unwired: 8 in]
      }
      frame "LaunchConfigDialog" {
        n160 = call "Launch XY Config Dialog.vi"("error in (no error)"=w454, "Waveform Graph Data in"=w451) -> ("error out"=w453:errorcluster)  [unwired: 9 in]
      }
      frame "Validate Channels" {
        n161 = Unbundle By Name(w460) -> ("System.Root"=w458:refnum<k24>, "Persistent Data.UDP Data.Channel Paths"=w456:string[])
        n162 = call "Validate Channels.vi"("Channel Paths"=w456, "Root"=w458) -> ("Valid Channels?"=w457:bool)  [unwired: 9 in]
        n163 = Bundle By Name(cluster=w460, "System.Valid Channels?"=w457) -> (w459:T10)
      }
      frame "Delete" {
        n164 = Unbundle By Name(w469) -> ("System.To Workspace"=w467:refnum<user-event>)
        n165 = Bundle By Name(cluster=T26 {"Operation"=enum."DeleteItem", "Data"=variant} ("event data"), "Operation"=enum16{"SetCustomData", "DeleteItem"}."DeleteItem") -> (w464:T26)
        n166 = Generate User Event(user event=w467, event data cluster=w464, error in=w468) -> (error out=w466:errorcluster)  [unwired: 1 in, 1 out]
      }
      frame "<------------- UDP Streaming ------------->" {
      }
      frame "Change Update Rate" {
        n167 = Unbundle By Name(w483) -> ("System.Graph Update Queue"=w478:refnum<queue>, "Persistent Data.UDP Data.Update Rate"=w476:T20)
        n168 = Index Array(array=u32[] [67, 100, 200, 250, 333, 500, 1000, 2000], index=w476) -> (element=w473:u32)
        n169 = To Variant(anything=w473) -> (Variant=w480:variant)
        n170 = Bundle By Name(cluster=T8 {"Graph Update Action State"=enum."Active", "Data"=variant} ("notification"), "Graph Update Action State"=Graph_Update_Action_State."Change Rate", "Data"=w480) -> (w479:T8)
        n171 = Enqueue Element At Opposite End(queue=w478, element=w479, error in (no error)=w475) -> (error out=w474:errorcluster)  [unwired: 1 in, 2 out]
      }
      frame "<------------- Front Panel Updates------------->" {
      }
      frame "Set Label" {
        n172 = Unbundle By Name(w489) -> ("Persistent Data.Label"=→"Label":string)
      }
      frame "Set Autoscale X" {
        # "If autoscale was turned off, save the current range"
        # "Make sure the button value is consistent in case this was set at start up or by the dialog"
        n173 = Unbundle By Name(w501) -> ("References.X.Scale.Once"=w493:refnum<vi>, "References.X.Scale.Auto"=w503:refnum<vi>, "References.Graph"=w507:refnum<vi>, "Persistent Data.Graph Props.Scale Properties.X.Auto"=w495:bool)
        "X.Autoscale" <- w495
        n174 = Select(t=u8 2 ("X Scale.Scale Fit"), s=w495, f=u8 0 ("X Scale.Scale Fit")) -> (s? t:f=w504:u8)
        n175 = property on="Property Node" class="XYGraph (strict)"(reference=w507, error in=w508, "XScale.ScaleFit"=w504) -> (error out=w502:errorcluster, "XScale.Minimum"=w499:dbl, "XScale.Maximum"=w498:dbl)  [unwired: 1 out]
        n176 = Build Array(w493) -> (w492:refnum<vi>[])
        n177 = case shown="True" w495 {
          tunnel: w501 -> [w513 w514]
          tunnel: [w512 w514] -> w500
          tunnel: w499 -> [w511 _]
          tunnel: w498 -> [w510 _]
          frame False {
            n178 = Bundle By Name(cluster=w513, "Persistent Data.Graph Props.Scale Properties.X.Min"=w511, "Persistent Data.Graph Props.Scale Properties.X.Max"=w510) -> (w512:T10)
          }
          frame True {
          }
        }
        n179 = property on="Property Node" class="Bool (strict)"(reference=w503, error in=w502, "Value"=w495) -> (error out=w496:errorcluster)  [unwired: 1 out]
        n180 = Not(x=w495) -> (.not. x?=w494:bool)
        n181 = call "XY Set Control Enable State.vi"("error in (no error)"=w496, "Enabled?"=w494, "Controls"=w492) -> ("error out"=w497:errorcluster)  [unwired: 8 in]
      }
      frame "Set Autoscale Y" {
        # "If autoscale was turned off, save the current range"
        # "Make sure the button value is consistent in case this was set at start up or by the dialog"
        n182 = Unbundle By Name(w524) -> ("References.Y.Scale.Once"=w516:refnum<vi>, "References.Y.Scale.Auto"=w526:refnum<vi>, "References.Graph"=w530:refnum<vi>, "Persistent Data.Graph Props.Scale Properties.Y.Auto"=w517:bool)
        "Y.Autoscale" <- w517
        n183 = Select(t=u8 2 ("X Scale.Scale Fit"), s=w517, f=u8 0 ("X Scale.Scale Fit")) -> (s? t:f=w527:u8)
        n184 = property on="Property Node" class="XYGraph (strict)"(reference=w530, error in=w531, "YScale.ScaleFit"=w527) -> (error out=w525:errorcluster, "YScale.Minimum"=w522:dbl, "YScale.Maximum"=w521:dbl)  [unwired: 1 out]
        n185 = Build Array(w516) -> (w515:refnum<vi>[])
        n186 = case shown="True" w517 {
          tunnel: w524 -> [w536 w537]
          tunnel: [w535 w537] -> w523
          tunnel: w522 -> [w534 _]
          tunnel: w521 -> [w533 _]
          frame False {
            n187 = Bundle By Name(cluster=w536, "Persistent Data.Graph Props.Scale Properties.Y.Min"=w534, "Persistent Data.Graph Props.Scale Properties.Y.Max"=w533) -> (w535:T10)
          }
          frame True {
          }
        }
        n188 = property on="Property Node" class="Bool (strict)"(reference=w526, error in=w525, "Value"=w517) -> (error out=w520:errorcluster)  [unwired: 1 out]
        n189 = Not(x=w517) -> (.not. x?=w518:bool)
        n190 = call "XY Set Control Enable State.vi"("error in (no error)"=w520, "Enabled?"=w518, "Controls"=w515) -> ("error out"=w519:errorcluster)  [unwired: 8 in]
      }
      frame "Set BGColor" {
        n191 = Unbundle By Name(w541) -> ("References.Graph"=w540:refnum<vi>, "Persistent Data.Graph Props.BgColor"=w538:u32)
        n192 = property on="Property Node" class="XYGraph (strict)"(reference=w540, error in=w542, "BG Color"=w538) -> (error out=w539:errorcluster)  [unwired: 1 out]
      }
      frame "Set X&Y Format & Precision" {
        n193 = Unbundle By Name(w553) -> ("Persistent Data.Graph Props.Scale Properties.Y.Format"=w552:T18, "Persistent Data.Graph Props.Scale Properties.Y.Precision:"=w551:T17, "References.Graph"=w548:refnum<vi>, "Persistent Data.Graph Props.Scale Properties.X.Format"=w544:T18, "Persistent Data.Graph Props.Scale Properties.X.Precision"=w545:T17)
        n194 = case shown="Default" w544 {
          selector: w544 -> [w557 _]
          tunnel: w549 -> [w560 w564]
          tunnel: w548 -> [w559 w563]
          tunnel: [w558 w565] -> w546
          tunnel: w545 -> [w556 _]
          tunnel: [w555 w561] -> w547
          frame Default {
            n195 = property on="Property Node" class="XYGraph (strict)"(reference=w559, error in=w560, "XScale.Format"=w557, "XScale.Precision"=w556) -> (reference out=w555:refnum<vi>, error out=w558:errorcluster)
          }
          frame 9 {
            # "9: Auto format is not writable. Rather it means a format string is applied"
            n196 = property on="Property Node" class="XYGraph (strict)"(reference=w563, error in=w564, "XScale.FormatString"="%#_g" ("X Scale.Format String")) -> (reference out=w561:refnum<vi>, error out=w565:errorcluster)
          }
        }
        n197 = case shown="Default" w552 {
          selector: w552 -> [w567 _]
          tunnel: w546 -> [w570 w573]
          tunnel: w547 -> [w569 w572]
          tunnel: [w568 w574] -> w550
          tunnel: w551 -> [w566 _]
          frame Default {
            n198 = property on="Property Node" class="XYGraph (strict)"(reference=w569, error in=w570, "YScale.Format"=w567, "YScale.Precision"=w566) -> (error out=w568:errorcluster)  [unwired: 1 out]
          }
          frame 9 {
            # "9: Auto format is not writable. Rather it means a format string is applied"
            n199 = property on="Property Node" class="XYGraph (strict)"(reference=w572, error in=w573, "YScale.FormatString"="%#_g" ("X Scale.Format String")) -> (error out=w574:errorcluster)  [unwired: 1 out]
          }
        }
      }
      frame "Set X&Y Max & Min" {
        # "Dont set range if auto scale is on."
        n200 = Unbundle By Name(w585) -> ("References.Graph"=w584:refnum<vi>, "Persistent Data.Graph Props.Scale Properties.X.Auto"=w579:bool, "Persistent Data.Graph Props.Scale Properties.X.Max"=w583:dbl, "Persistent Data.Graph Props.Scale Properties.X.Min"=w582:dbl, "Persistent Data.Graph Props.Scale Properties.Y.Auto"=w577:bool, "Persistent Data.Graph Props.Scale Properties.Y.Max"=w576:dbl, "Persistent Data.Graph Props.Scale Properties.Y.Min"=w575:dbl)
        n201 = case shown="False" w579 {
          tunnel: w586 -> [w599 w600]
          tunnel: w584 -> [w598 w601]
          tunnel: w583 -> [w597 _]
          tunnel: w582 -> [w596 _]
          tunnel: [w595 w600] -> w581
          tunnel: [w594 w601] -> w580
          frame False {
            n202 = property on="Property Node" class="XYGraph (strict)"(reference=w598, error in=w599, "XScale.Maximum"=w597, "XScale.Minimum"=w596) -> (reference out=w594:refnum<vi>, error out=w595:errorcluster)
          }
          frame True {
          }
        }
        n203 = case shown="False" w577 {
          tunnel: w581 -> [w592 w593]
          tunnel: w580 -> [w591 _]
          tunnel: [w590 w593] -> w578
          tunnel: w576 -> [w589 _]
          tunnel: w575 -> [w588 _]
          frame False {
            n204 = property on="Property Node" class="XYGraph (strict)"(reference=w591, error in=w592, "YScale.Maximum"=w589, "YScale.Minimum"=w588) -> (error out=w590:errorcluster)  [unwired: 1 out]
          }
          frame True {
          }
        }
      }
      frame "Set Axis Labels" {
        n205 = Unbundle By Name(w619) -> ("System.Root"=w602:refnum<k24>, "Persistent Data.UDP Data.Channel Paths"=w607:string[], "Persistent Data.UDP Data.Channel Names"=w604:string[], "References.Graph"=w618:refnum<vi>, "Persistent Data.Graph Props.Scale Properties.X.DefLabel"=w614:bool, "Persistent Data.Graph Props.Scale Properties.X.Label:"=w613:string, "Persistent Data.Graph Props.Scale Properties.X.LabelVis"=w615:bool, "Persistent Data.Graph Props.Scale Properties.Y.DefLabel"=w610:bool, "Persistent Data.Graph Props.Scale Properties.Y.Label:"=w609:string, "Persistent Data.Graph Props.Scale Properties.Y.LabelVis"=w612:bool)
        n206 = Index Array(array=w607) -> (element=w605:string)  [unwired: 1 in]
        n207 = Index Array(array=w604) -> (element=w603:string)  [unwired: 1 in]
        n208 = Select(t="Amplitude", s=w610, f=w609) -> (s? t:f=w608:string)
        n209 = call "Get Channel Name.vi"("Channel Name"=w603, "Channel Path"=w605, "Root"=w602) -> ("Name"=w606:string)  [unwired: 8 in]
        n210 = Select(t=w606, s=w614, f=w613) -> (s? t:f=w616:string)
        n211 = property on="Property Node" class="XYGraph (strict)"(reference=w618, error in=w620, "XScale.NameLbl.Text"=w616, "XScale.NameLbl.Visible"=w615, "YScale.NameLbl.Text"=w608, "YScale.NameLbl.Visible"=w612) -> (error out=w617:errorcluster)  [unwired: 1 out]
      }
      frame "Set Legend" {
        n212 = Unbundle By Name(w636) -> ("System.Root"=w622:refnum<k24>, "Persistent Data.UDP Data.Channel Paths"=w628:string[], "Persistent Data.UDP Data.Channel Names"=w624:string[], "References.Graph"=w630:refnum<vi>, "Persistent Data.Graph Props.Legend:Visible"=w629:bool)
        n213 = Array Subset(array=w628, index=1) -> (w627:string[])  [unwired: 1 in]
        n214 = Array Subset(array=w624, index=1) -> (w623:string[])  [unwired: 1 in]
        n215 = Array Size(array=w627) -> (size(s)=w632:i32)
        n216 = property class="XYGraph (strict)"(reference=w630, error in=w634, "LegNumRows"=w632, "Legend Visible"=w629) -> (reference out=w631:refnum<vi>, error out=w633:errorcluster)
        n217 = case shown="Default" w632 {
          tunnel: [w643 w657] -> w635
          tunnel: w633 -> [w642 w653]
          tunnel: w627 -> [w641 _]
          tunnel: w631 -> [w640 w654]
          tunnel: w623 -> [w639 _]
          tunnel: w622 -> [w638 _]
          frame Default {
            n218 = for {
              shift-right: [w650] -> w643
              shift-left: w642 -> [w651]
              tunnel: w641 -> [w647] mode=indexing
              tunnel: w640 -> [w648]
              tunnel: w639 -> [w645] mode=indexing
              tunnel: w638 -> [w644]
              i -> [w649]
              n219 = call "Get Channel Name.vi"("Channel Name"=w645, "Channel Path"=w647, "Root"=w644) -> ("Name"=w646:string)  [unwired: 8 in]
              n220 = property class="XYGraph (strict)"(reference=w648, error in=w651, "Active Plot"=w649, "Plot.Plot Name"=w646) -> (error out=w650:errorcluster)  [unwired: 1 out]
            }
          }
          frame 0 {
            # "If there are no streams this is a good opportunity to clear the graph"
            n221 = property class="XYGraph (strict)"(reference=w654, error in=w653, "Active Plot"=u32 0, "Plot.Plot Name"="Plot 0", "Value"=cluster{"X":dbl[], "Y":dbl[]}[] []) -> (error out=w657:errorcluster)  [unwired: 1 out]
          }
        }
      }
      frame "<------------------ Shut Down ------------------>" {
      }
      frame "Delete Events" {
        # "These nodes run even if error occures"
        n222 = Unbundle By Name(w686) -> ("System.ToDialog"=w670:refnum<user-event>, "System.DialogEventReg"=w672:refnum<event-registration>, "System.Update Graph"=w663:refnum<user-event>, "System.Periodic"=w673:refnum<user-event>, "System.FromDialog"=w677:refnum<user-event>, "System.To Workspace"=w684:refnum<user-event>, "System.From Workspace"=w685:refnum<user-event>, "EventRegs.Graph"=w682:refnum<event-registration>, "System.SystemStateRefs"=w679:T22, "System.Graph Update Queue"=w666:refnum<queue>, "System.UDP Queue"=w665:refnum<queue>)
        n223 = call <vilib>:"NI VeriStand - Close Engine State Change Notification.vi"("SystemStateRefs"=w679) -> ("error out"=w675:errorcluster)  [unwired: 10 in]
        n224 = Release Queue(queue=w666) -> (error out=w667:errorcluster)  [unwired: 2 in, 2 out]
        n225 = Release Queue(queue=w665) -> (error out=w664:errorcluster)  [unwired: 2 in, 2 out]
        n226 = Unregister For Events(event registration refnum=w682) -> (error out=w681:errorcluster)  [unwired: 1 in]
        n227 = Destroy User Event(user event=w685, error in=w681) -> (error out=w680:errorcluster)
        n228 = Destroy User Event(user event=w684, error in=w680) -> (error out=w678:errorcluster)
        n229 = Destroy User Event(user event=w677, error in=w678) -> (error out=w674:errorcluster)
        n230 = Destroy User Event(user event=w673, error in=w674) -> (error out=w661:errorcluster)
        n231 = Destroy User Event(user event=w663, error in=w661) -> (error out=w662:errorcluster)
        n232 = Unregister For Events(event registration refnum=w672) -> (error out=w671:errorcluster)  [unwired: 1 in]
        n233 = Destroy User Event(user event=w670, error in=w671) -> (error out=w668:errorcluster)
        n234 = Merge Errors(w669, w668, w662, w675, w667, w664) -> (w676:errorcluster)
      }
      frame "Close Managers" {
        # "These nodes run even if error occures"
        n235 = Unbundle By Name(w689) -> ("System.Workspace"=w688:T21)
        n236 = call <vilib>:"NI VeriStand - Close Workspace Manager Reference.vi"("error in (no error)"=w690, "WorkspaceManager"=w688) -> ("error out"=w687:errorcluster)  [unwired: 9 in]
      }
      frame "Wait for NIVS Helper" {
        # "This node runs even if error occures"
        # "Wait for the NIVS helper VI to finish"
        n237 = Unbundle By Name(w700) -> ("System.NIVS helper"=w699:refnum<vi>)
        n238 = call-by-ref "Wait On Asynchronous Call"(reference=w699) -> (reference out=w695:refnum<vi>, error out=w698:errorcluster, 19:"error out"=w697:errorcluster)  [unwired: 20 in]
        n239 = Merge Errors(w698, w697) -> (w696:errorcluster)
        n240 = Close Reference(reference=w695, error in (no error)=w696) -> (error out=w692:errorcluster)
        n241 = Merge Errors(w694, w692) -> (w693:errorcluster)
      }
      frame "Exit" {
      }
      frame "<------------------ Macros ------------------>" {
      }
      frame "MACRO - Initialize" {
        # "Save persistent data at the end so we can detect if this control is new or not after next load"
        n242 = Build Array (concatenate)(string[] ["Open Managers", "Create Events", "Get Control References", "Get Persistent Data", "Validate Channels", "Check Connection", "Initialize Plots & Legend", "MACRO - Refresh Graph", "Launch NIVS Helper", "Save Persistent Data"], w710) -> (w709:string[])
      }
      frame "MACRO - Shut Down" {
        n243 = Build Array (concatenate)(string[] ["Delete Events", "Close Managers", "Wait for NIVS Helper", "Exit"], w717) -> (w716:string[])
      }
      frame "MACRO - Refresh Graph" {
        n244 = Build Array (concatenate)(string[] ["Change Update Rate", "Set Label", "Set X&Y Max & Min", "Set Autoscale X", "Set Autoscale Y", "Set BGColor", "Set X&Y Format & Precision", "Set Axis Labels", "Set Legend"], w723) -> (w720:string[])
      }
      frame "MACRO - Disconnect" {
        n245 = Build Array (concatenate)(string[] ["Close UDP Streaming"], w726) -> (w725:string[])
      }
      frame "MACRO - System Disconnect" {
        n246 = Build Array (concatenate)(string[] ["System Close UDP Streaming"], w731) -> (w730:string[])
      }
      frame "MACRO - Connect" {
        n247 = Build Array (concatenate)(string[] ["Save Persistent Data", "Change Update Rate", "Open UDP Streaming"], w738) -> (w735:string[])
      }
      frame "<----------------- Disconnect ------------------->" {
      }
      frame "Close UDP Streaming" {
        n248 = Unbundle By Name(w753) -> ("System.UDPChannelStreamSession"=w747:T23, "System.Graph Update Queue"=w755:refnum<queue>, "System.UDP Queue"=w756:refnum<queue>)
        n249 = Enqueue Element(queue=w756, element=T9 {"UDP Action State"=enum."Close", "Data"=variant} ("notification"), error in (no error)=w754) -> (error out=w746:errorcluster)  [unwired: 1 in, 2 out]
        n250 = Enqueue Element(queue=w755, element=T8 {"Graph Update Action State"=enum."Inactive", "Data"=variant} ("notification"), error in (no error)=w746) -> (error out=w745:errorcluster)  [unwired: 1 in, 2 out]
        n251 = call <vilib>:"NI VeriStand - Undeploy UDP Channel Streaming Session.vi"("error in (no error)"=w745, "UDPChannelStreamSession in"=w747) -> ("error out"=w744:errorcluster, "UDPChannelStreamSession out"=w742:T23)  [unwired: 8 in]
        n252 = Bundle By Name(cluster=w753, "UDP Stream Active?"=FALSE, "System.UDPChannelStreamSession"=T23 refnum) -> (w752:T10)
        n253 = call <vilib>:"NI VeriStand - Close UDP Channel Streaming Session.vi"("error in (no error)"=w744, "UDPChannelStreamSession in"=w742) -> ("error out"=w743:errorcluster)  [unwired: 9 in]
      }
      frame "System Close UDP Streaming" {
        n254 = Unbundle By Name(w767) -> ("System.UDPChannelStreamSession"=w759:T23, "System.Graph Update Queue"=w769:refnum<queue>, "System.UDP Queue"=w770:refnum<queue>)
        n255 = Enqueue Element(queue=w770, element=T9 {"UDP Action State"=enum."Close", "Data"=variant} ("notification"), error in (no error)=w768) -> (error out=w761:errorcluster)  [unwired: 1 in, 2 out]
        n256 = Enqueue Element(queue=w769, element=T8 {"Graph Update Action State"=enum."Inactive", "Data"=variant} ("notification"), error in (no error)=w761) -> (error out=w758:errorcluster)  [unwired: 1 in, 2 out]
        n257 = Bundle By Name(cluster=w767, "UDP Stream Active?"=FALSE, "System.UDPChannelStreamSession"=T23 refnum) -> (w766:T10)
        n258 = call <vilib>:"NI VeriStand - Close UDP Channel Streaming Session.vi"("error in (no error)"=w758, "UDPChannelStreamSession in"=w759) -> ("error out"=w760:errorcluster)  [unwired: 9 in]
      }
      frame "<----------------- Connect ------------------->" {
      }
      frame "Open UDP Streaming" {
        n259 = Unbundle By Name(w793) -> ("System.Workspace"=w797:T21, "System.Graph Update Queue"=w788:refnum<queue>, "System.UDP Queue"=w791:refnum<queue>, "Persistent Data.UDP Data"=w776:T19, "System.Root"=w790:refnum<k24>, "Persistent Data.UDP Data.History Length"=w787:dbl, "Persistent Data.UDP Data.Decimation"=w785:i32)
        n260 = call "Get UDP Buffer Size.vi"("Decimation"=w785, "History Length"=w787, "Root"=w790) -> ("Buffer Size"=w784:i32)  [unwired: 8 in]
        n261 = call "Init UDP Config.vi"("error in (no error)"=w796, "Graph Buffer Size"=w784, "UDP Data"=w776, "Workspace anager in"=w797) -> ("error out"=w781:errorcluster, "UDP Stream Configuration"=w778:T5, "UDPChannelStreamSession out"=w794:T23, "WorkspaceManager out"=w795:T21)  [unwired: 4 in]
        n262 = To Variant(anything=w778) -> (Variant=w777:variant)
        n263 = Bundle By Name(cluster=T9 {"UDP Action State"=enum."Idle", "Data"=variant} ("notification"), "UDP Action State"=UDP_Action_State."Open", "Data"=w777) -> (w779:T9)
        n264 = Enqueue Element(queue=w791, element=w779, error in (no error)=w781) -> (error out=w786:errorcluster)  [unwired: 1 in, 2 out]
        n265 = Bundle By Name(cluster=w793, "System.Workspace"=w795, "System.UDPChannelStreamSession"=w794, "UDP Stream Active?"=TRUE) -> (w792:T10)
        n266 = Enqueue Element(queue=w788, element=T8 {"Graph Update Action State"=enum."Active", "Data"=variant} ("notification"), error in (no error)=w786) -> (error out=w789:errorcluster)  [unwired: 1 in, 2 out]
      }
      frame "<------------------ Initialization ------------------>" {
      }
      frame "Open Managers" {
        n267 = Unbundle By Name(w804) -> ("System.Gtwy"=w803:string)
        n268 = call <vilib>:"NI VeriStand - Open Workspace Manager Reference.vi"("error in (no error)"=w807, "Gateway IP Address (\"\": localhost)"=w803) -> ("error out"=w802:errorcluster, "WorkspaceManager"=w805:T21)  [unwired: 8 in]
        n269 = Bundle By Name(cluster=w804, "System.Workspace"=w805) -> (w806:T10)
      }
      frame "Create Events" {
        n270 = call "Create XY Events.vi"("error in (no error)"=w810, "Waveform Graph Data in"=w809) -> ("error out"=w812:errorcluster, "Waveform Graph Data out"=w813:T10)  [unwired: 8 in]
      }
      frame "Get Control References" {
        n271 = control-ref of="Graph"() -> (w814:refnum<vi>)
        n272 = control-ref of="X.Scale.Auto"() -> (w818:refnum<vi>)
        n273 = control-ref of="Y.Scale.Auto"() -> (w819:refnum<vi>)
        n274 = control-ref of="X.Scale.Once"() -> (w817:refnum<vi>)
        n275 = control-ref of="Y.Scale.Once"() -> (w816:refnum<vi>)
        n276 = control-ref of="Legend"() -> (w815:refnum<vi>)
        n277 = Bundle By Name(cluster=w822, "References.Graph"=w814, "References.X.Scale.Auto"=w818, "References.Y.Scale.Auto"=w819, "References.X.Scale.Once"=w817, "References.Y.Scale.Once"=w816, "References.LegendVis"=w815) -> (w821:T10)
      }
      frame "Get Persistent Data" {
        # "True if this is a brand new control. Used by the from workspace event"
        n278 = Unbundle By Name(w831) -> ("Custom Data"=w832:variant)
        n279 = call "XY Variant to Persistent Data.vi"("error in (no error)"=w834, "Variant"=w832) -> ("error out"=w833:errorcluster, "Persistent Data"=w824:T13, "New"=w828:bool)  [unwired: 7 in]
        n280 = Build Array (concatenate)("Initialize Dialog", w829) -> (w826:string[])
        n281 = Select(t=w826, s=w828, f=w829) -> (s? t:f=w825:string[])
        n282 = Bundle By Name(cluster=w831, "System.New"=w828, "Persistent Data"=w824) -> (w830:T10)
      }
      frame "Initialize Dialog" {
        n283 = Bundle By Name(cluster=w838, "Persistent Data.UDP Data"=T19 {"Decimation"=1, "UDP Buffer Size"=8192, "History Length"=10.0, "Update Rate"=enum."5 Hz", "Channel Paths"=[], "Channel Names"=[]}, "System.Valid Channels?"=FALSE) -> (w837:T10)
      }
      frame "Check Connection" {
        w850 = T30 1 items=["Idle", "Active"] ("x")
        # "This only needs to be done at start up because while running we will get the system state change event"
        n284 = Unbundle By Name(w844) -> ("System.Valid Channels?"=w841:bool, "System.Workspace"=w852:T21)
        n285 = call <vilib>:"NI VeriStand - Get System State.vi"("error in (no error)"=w854, "WorkspaceManager in"=w852) -> ("error out"=w853:errorcluster, "System State"=w851:T30)  [unwired: 5 in, 3 out]
        n286 = Equal?(x=w850, y=w851) -> (x = y?=w842:bool)
        n287 = Bundle By Name(cluster=w844, "System.Connected?"=w842) -> (w845:T10)
        n288 = And(x=w841, y=w842) -> (x .and. y?=w843:bool)
        n289 = case shown="True" w843 {
          tunnel: [w856 w862] -> w849
          tunnel: w848 -> [w856 w861]
          tunnel: "MACRO - Connect" -> [_ w860]
          tunnel: [w855 w857] -> w846
          tunnel: w845 -> [w855 w859]
          frame False {
          }
          frame True {
            # "If we are connecting at start up... use the plot width that we last saved. This prevents weird behavior because NIVS might be resizing our widget  during workspace initialization."
            n290 = Bundle By Name(cluster=w859, "System.UseSavedWidth"=TRUE) -> (w857:T10)
            n291 = Build Array (concatenate)(w860, w861) -> (w862:string[])
          }
        }
      }
      frame "Initialize Plots & Legend" {
        n292 = Unbundle By Name(w872) -> ("References.LegendVis"=w866:refnum<vi>, "Persistent Data.Graph Props.Legend:Visible"=w865:bool, "References.Graph"=w863:refnum<vi>, "Persistent Data.Graph Props.Plots"=w870:T15[], "Persistent Data.Graph Props.Legend:Number of Rows"=w869:u32)
        n293 = call "Update XY Plots.vi"("error in (no error)"=w871, "Persistent Data.Graph Props.Legend:Number of Rows"=w869, "Plots"=w870, "Graph"=w863) -> ("error out"=w868:errorcluster)  [unwired: 7 in]
        n294 = Not(x=w865) -> (.not. x?=w864:bool)
        n295 = property class="Bool (strict)"(reference=w866, error in=w868, "Value"=w864) -> (error out=w867:errorcluster)  [unwired: 1 out]
      }
      frame "Launch NIVS Helper" {
        # "This VI is required to be run to connect this workspace object to the workspace. This VI will continue to run until this control is deleted or the workspace is closed. Therefore, launch it asynchronously so there is no need for a separate loop."
        n296 = Unbundle By Name(w881) -> ("System.From Workspace"=w879:refnum<user-event>, "System.To Workspace"=w878:refnum<user-event>)
        n297 = vi-ref <vilib>:"sub_Display Template Handler Custom.vi"() -> (w886:refnum<vi>)
        n298 = property class="VI"(reference=w886, error in=w887) -> (error out=w885:errorcluster, "Name"=w884:string)  [unwired: 1 out]
        n299 = Current VI's Path() -> (path=w880:path)
        n300 = Open VI Reference(type specifier VI Refnum (for type only)=refnum<vi> refnum, vi path=w884, options=256, error in (no error)=w885) -> (vi reference=w882:refnum<vi>, error out=w889:errorcluster)  [unwired: 2 in]
        n301 = call-by-ref "Start Asynchronous Call"(reference=w882, error in=w889, "Parent.Path"=w880, "ToWidgetEvent"=w879, "ToWorkspace"=w878, "Item.Data"=w877, "Resizable"=TRUE) -> (reference out=w874:refnum<vi>, error out=w888:errorcluster)  [unwired: 14 in, 1 out]
        n302 = Bundle By Name(cluster=w881, "System.NIVS helper"=w874) -> (w875:T10)
      }
    }
    n303 = Unbundle By Name(w124) -> ("System.ErrFlag"=w123:bool)
    n304 = Compound Arithmetic op=AND(invert w123, w121) -> (w122:bool)
    n305 = case shown="True" w122 {
      selector: w122 -> [_ w138]
      tunnel: w131 -> [w136 w141]
      tunnel: [w136 w142] -> w128
      tunnel: [w135 w139] -> w125
      tunnel: w124 -> [w135 w140]
      tunnel: w120 -> [_ w137]
      frame False {
      }
      frame True {
        n306 = Bundle By Name(cluster=w140, "System.ErrState"=w137, "System.ErrFlag"=w138) -> (w139:T10)
        n307 = Build Array (concatenate)("Error", w141) -> (w142:string[])
      }
    }
  }
  n308 = call <vilib>:"Simple Error Handler.vi"("error in (no error)"=w1) -> ()  [unwired: 4 in, 5 out]
